vi "From Variant.vi"(0 "Obj in":refnum<class "State.lvclass">, 7 "Variant":variant, 9 "Prefix":string, 11 "error in (no error)":errorcluster) -> (4 "Obj out":refnum<class "State.lvclass">, 15 "error out":errorcluster)   [LabVIEW 2020, in "State.lvclass"]
uses:
  State.lvclass
  State.lvclass/State.ctl
  epl-vi-lib/Koop/KObject Class/KObject.lvclass
  Timeout/Timeout.lvclass
  Termination/Termination.lvclass
  epl-vi-lib/Signal Synthesis VIs/4th Generation/Classes/SignalManager/SignalManager.lvclass
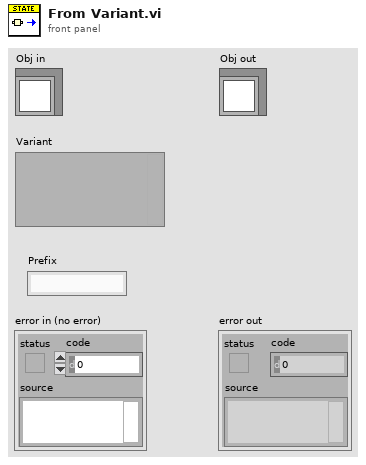
[diagram p1: front panel]
types:
  T1 = typedef "State.lvclass/Serialized.ctl" = cluster{"Name":string, "TTL-only":bool, "Timeouts":refnum<class "Timeout.lvclass">[], "Term":refnum<class "Termination.lvclass">[], "SigMan":refnum<class "SignalManager.lvclass">, "Grating":T2, "Execute script":bool}
  T2 = typedef "Tosca-Grating.ctl" = cluster{"Type":T3, "Orientation (deg)":dbl, "Spatial frequency (cpd)":dbl, "Velocity (Hz)":dbl, "Contrast":dbl, "Background intensity":dbl, "Duration (ms)":dbl, "Phase (cycles)":dbl}
  T3 = typedef "Tosca-Grating Type.ctl" = enum16{"OFF", "Square", "Sine"}
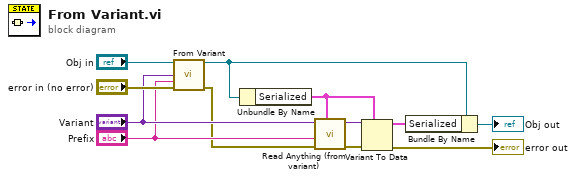
[diagram p0: block diagram]
diagram:
  n1 = call-parent "From Variant.vi"("KObject in"="Obj in", "Variant"="Variant", "Prefix"="Prefix", "error in (no error)"="error in (no error)") -> ("KObject out"=w3:refnum<class "State.lvclass">, "error out"=w4:errorcluster)  [unwired: 10 in]
  n2 = Unbundle By Name(w3) -> ("Serialized"=w8:T1)
  n3 = call "Read Anything (from variant).vi"("Type of Anything"=w8, "Error In"=w4, "Prefix"="Prefix", "Variant Database"="Variant") -> ("Error Out"=w9:errorcluster, "Anything"=w10:variant)  [unwired: 5 in, 1 out]
  n4 = Variant To Data(error in=w9, type=w8, Variant=w10) -> (data=w7:T1, error out=→"error out":errorcluster)
  n5 = Bundle By Name(cluster=w3, "Serialized"=w7) -> (→"Obj out":refnum<class "State.lvclass">)
